vi "Sort 2D String Array - String Transform (Post Sort).vi"(7 "Input String (\" \")":string) -> (8 "Output String (\" \")":string)   [LabVIEW 2009, in "xijk_select_best_filter.lvlib"]
doc: "Sort 2D String Array - StringTransform (Post Sort).vi\n\n<B>Description:</B>\n\nThis VI transforms strings that sorted properly using the sort 1D array function into strings representing numbers or text based on the content of the meta tag at the end of each string. \n\nIf the input string represents a number, this VI restores the number's original formatting based on the meta tag data. \n\nIf the input is a string, this VI restores the lexical class of each character in the string based on the meta tag data.\n\n<B>Usage:</B>\n\nWire all required inputs.\n\n<B>Inputs:</B>\n\nInput String\n- The string to transform.\n\n<B>Outputs:</B>\n\nOutput String\n- Description: This is the output string.\n\n<B>Developed by:</B>\n\nMark Ridgley\nmark.ridgley@logicpd.com"
uses:
  xijk_select_best_filter.lvlib
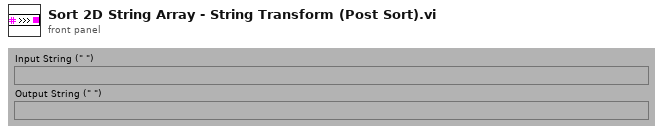
[diagram p1: front panel]
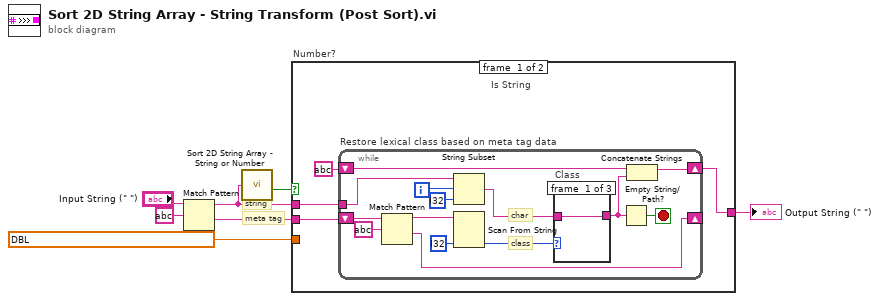
[diagram p0: block diagram]
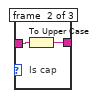
[diagram p2: hidden frame]
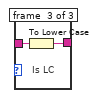
[diagram p3: hidden frame]
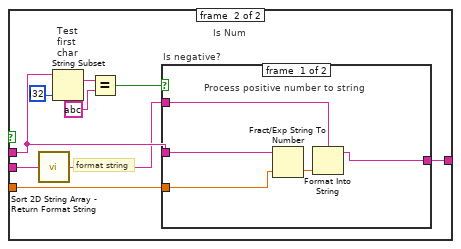
[diagram p4: hidden frame]
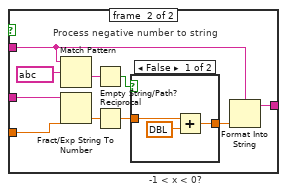
[diagram p5: hidden frame]
diagram:
  # "meta tag"
  # "string"
  n1 = Match Pattern(string="Input String (\" \")", regular expression=string ? ("search char (-)")) -> (before substring=w1:string, after substring=w3:string)  [unwired: 3 out]
  n2 = call "Sort 2D String Array - String or Number.vi"("Input String (\" \")"=w1) -> ("Is Num? (F)"=w2:bool)  [unwired: 14 out]
  n3 = case "Number?" shown="True" w2 {
    tunnel: [w9 w39] -> w7
    tunnel: w1 -> [w11 w38]
    tunnel: w3 -> [w8 w32]
    tunnel: dbl ? ("default (0 dbl)") -> [_ w33]
    frame #0 {
      # "Is String"
      n4 = while "Restore lexical class based on meta tag data" {
        tunnel: w11 -> [w25]
        shift-right: [w18] -> w9
        shift-left: string ? -> [w17]
        shift-right: [w12] -> _
        shift-left: w8 -> [w22]
        i -> [w24]
        stop <- w15 stop-if-true
        # "char"
        # "class"
        n5 = Match Pattern(string=w22, regular expression=string ? ("search string/char (-)")) -> (before substring=w13:string, after substring=w12:string)  [unwired: 3 out]
        n6 = String Subset(string=w25, offset (0)=w24, length (rest)=i32 ? ("length (rest)")) -> (substring=w16:string)
        n7 = Scan From String(input string=w13, default 1=i32 ? ("length (rest)")) -> (output 1=w19:i32)  [unwired: 3 in, 3 out]
        n8 = case "Class" shown="4" w19 {
          tunnel: w16 -> [w26 w28 w30]
          tunnel: [w26 w27 w29] -> w14
          frame #0 {
          }
          frame #1 {
            # "Is cap"
            n9 = To Upper Case(1:w28) -> (0:w27:string)
          }
          frame #2 {
            # "Is LC"
            n10 = To Lower Case(string=w30) -> (all lower case string=w29:string)
          }
        }
        n11 = Empty String/Path?(string/path=w14) -> (empty?=w15:bool)
        n12 = Concatenate Strings(w17, w14) -> (w18:string)
      }
    }
    frame #1 {
      # "format string"
      # "Is Num"
      n13 = call "Sort 2D String Array - Return Format String.vi"("Input String (\" \")"=w32) -> ("Format String"=w31:string)  [unwired: 14 out]
      n14 = String Subset "Test\nfirst\nchar"(string=w38, length (rest)=i32 ? ("offset (0)")) -> (substring=w37:string)  [unwired: 1 out]
      n15 = Equal?(x=w37, y=string ?) -> (x = y?=w35:bool)
      n16 = case "Is negative?" shown="True" w35 {
        tunnel: [w43 w54] -> w39
        tunnel: w38 -> [w42 w50]
        tunnel: w31 -> [w41 w45]
        tunnel: w33 -> [w40 w46]
        frame #0 {
          # "Process positive number to string"
          n17 = Fract/Exp String To Number(string=w42, default (0 dbl)=w40) -> (number=w44:dbl)  [unwired: 3 out]
          n18 = Format Into String(format string=w41, w44) -> (resulting string=w43:string)  [unwired: 2 in, 1 out]
        }
        frame #1 {
          # "Process negative number to string"
          n19 = Match Pattern(string=w45, regular expression=string ? ("search char (-)")) -> (after substring=w47:string)  [unwired: 4 out]
          n20 = Fract/Exp String To Number(string=w50, default (0 dbl)=w46) -> (number=w53:dbl)  [unwired: 3 out]
          n21 = Empty String/Path?(string/path=w47) -> (empty?=w48:bool)
          n22 = Reciprocal(x=w53) -> (1/x=w52:dbl)
          n23 = case "-1 < x < 0?" shown="False" w48 {
            tunnel: w52 -> [w57 w58]
            tunnel: [w56 w58] -> w51
            frame #0 {
              n24 = Add(x=w57, y=dbl ?) -> (x+y=w56:dbl)
            }
            frame #1 {
            }
          }
          n25 = Format Into String(format string=w45, w51) -> (resulting string=w54:string)  [unwired: 2 in, 1 out]
        }
      }
    }
  }
  "Output String (\" \")" <- w7
